vi "Run Servo.vi"   [LabVIEW 2019]
uses:
  Robot Global Data.vi
types:
  T1 = typedef "WPI_ServoDeviceRef.ctl" = cluster{"DeviceStatus":errorcluster, "PWM Channel":T2, "DeadBand":T3}
  T2 = typedef "FPGA_DIOPWMChannel.ctl" = enum8{"PWM 0", "PWM 1", "PWM 2", "PWM 3", "PWM 4", "PWM 5", "PWM 6", "PWM 7", "PWM 8", "PWM 9", "PWM MXP 0", "PWM MXP 1", "PWM MXP 2", "PWM MXP 3", "PWM MXP 4", "PWM MXP 5", "PWM MXP 6", "PWM MXP 7", "PWM MXP 8", "PWM MXP 9", "Invalid"}
  T3 = typedef "WPI_PWMDeadband.ctl" = cluster{"Name":string, "maxPositivePwm":i32, "minPositivePwm":i32, "centerPwm":i32, "maxNegativePwm":i32, "minNegativePwm":i32, "angularRange":u16}
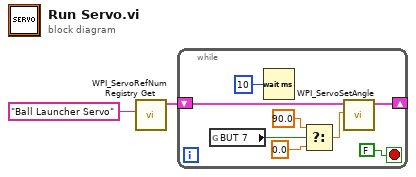
[diagram p0: block diagram]
diagram:
  n1 = call <vilib>:"WPI_ServoRefNum Registry Get.vi"("refnum name"="Ball Launcher Servo") -> ("ServoDeviceRef"=w1:T1)  [unwired: 9 in, 1 out]
  n2 = while {
    shift-right: [w6] -> _
    shift-left: w1 -> [w5]
    stop <- FALSE stop-if-true
    n3 = global read "Robot Global Data.vi" "BUT 7"() -> (w3:bool)
    n4 = Wait (ms)(milliseconds to wait=u32 10) -> ()  [unwired: 1 out]
    n5 = Select(t=90.0, s=w3, f=0.0) -> (s? t:f=w4:dbl)
    n6 = call <vilib>:"WPI_ServoSetAngle.vi"("Angle"=w4, "ServoDeviceRef"=w5) -> ("ServoDeviceRef"=w6:T1)  [unwired: 8 in, 1 out]
  }
